vi "TempScanPan.vi"(8 "error in (no error)":errorcluster caption="entrée d'erreur (pas d'erreur)", 11 "LSCI332.lvclass":refnum<class "LSCI332.lvclass">) -> (0 "error out":errorcluster caption="sortie d'erreur", 3 "LSCI332.lvclass Out":refnum<class "LSCI332.lvclass">)   [LabVIEW 2019, in "LSCI332.lvclass"]
uses:
  LSCI332.lvclass
  C:/Programmes Labview/LabScanV1A/DevicesClass/BaseDevice/BaseDevice.lvclass
  BaseDevice/Accessor/GetClassEvent.vi
panel:
  in  "ForceStop":bool
  in  "Wait Stab":bool=TRUE
  in  "Timeout":u32=600 caption="Timeout(s)"
  in  "InRangeTime":i32=300 caption="\"In Range\" Time(s)"
  in  "RangeK":dbl=1.0 min=0.01 max=100.0 step=0.01
  in  "MainProgQEvent":refnum<user-event>
  in  "MainProgQ":refnum<queue>
  in  "Acq":bool
  in  "Boucle(1)":u32(ring) caption="Boucle" items=["Boucle 1", "Boucle 2"]
  in  "Stop":bool
  in  "MiseAJour":bool
  out "Init Program":bool
  # "this MUST labeled with class name"
  # "this MUST be present and labeled \"Stop\""
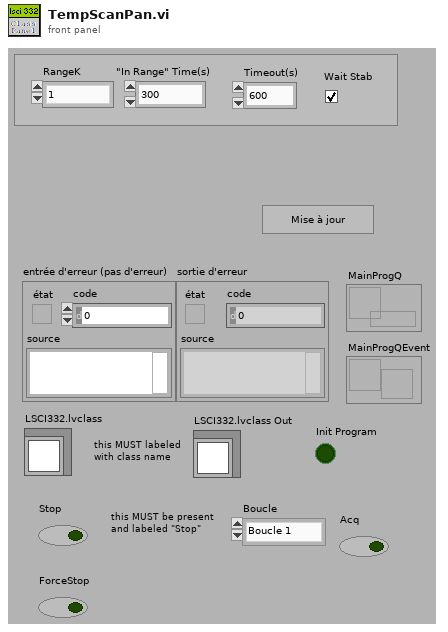
[diagram p1: front panel]
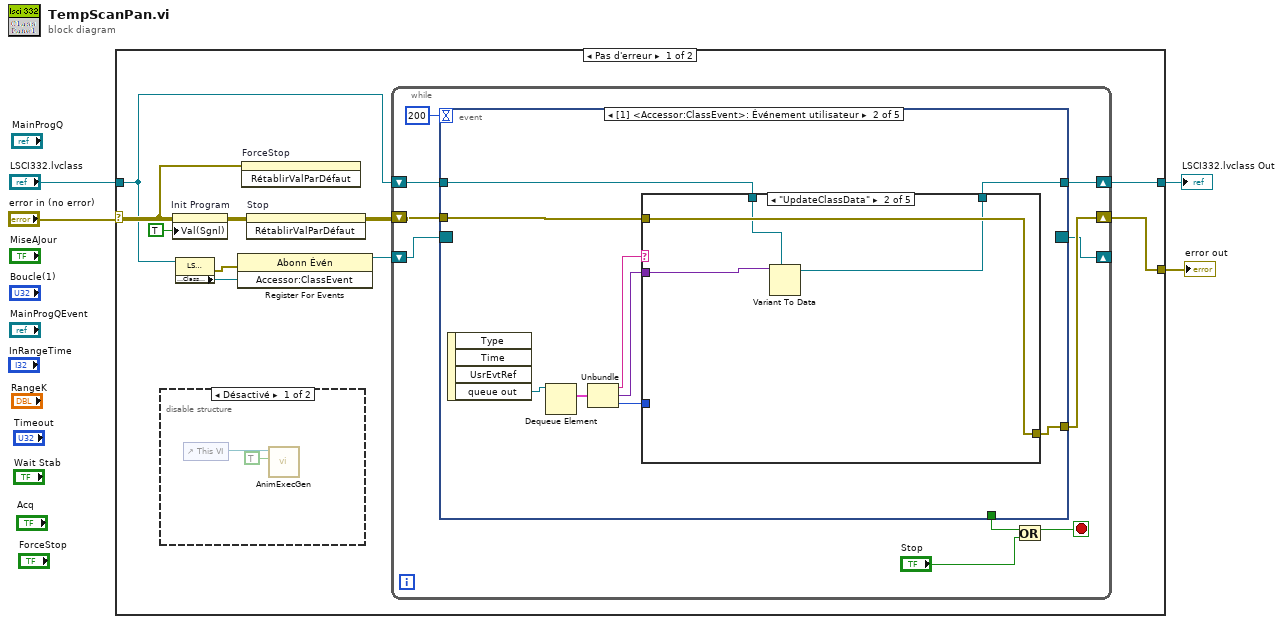
[diagram p0: block diagram]
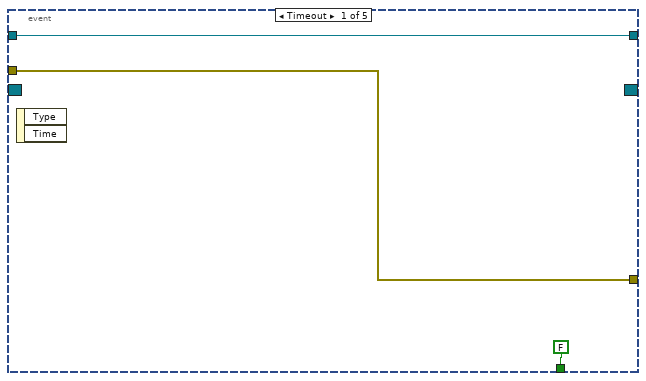
[diagram p3: hidden frame]
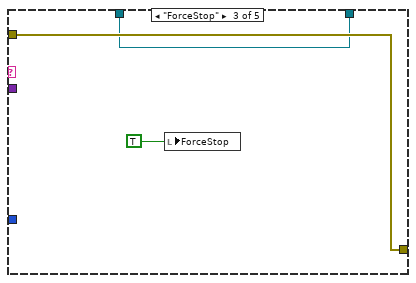
[diagram p5: hidden frame]
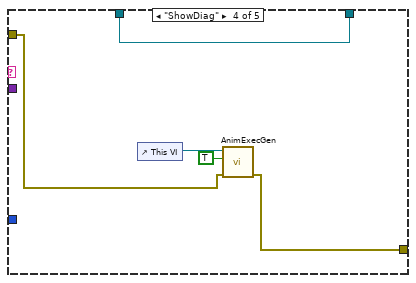
[diagram p6: hidden frame]
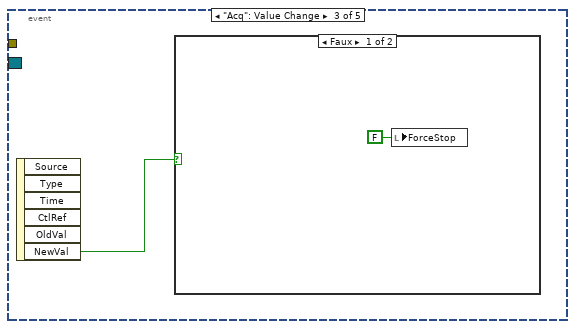
[diagram p8: hidden frame]
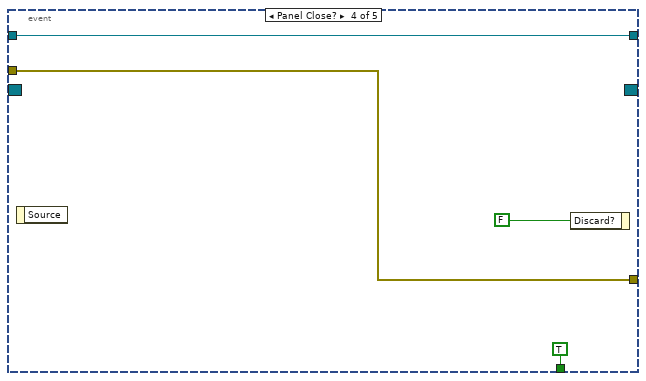
[diagram p10: hidden frame]
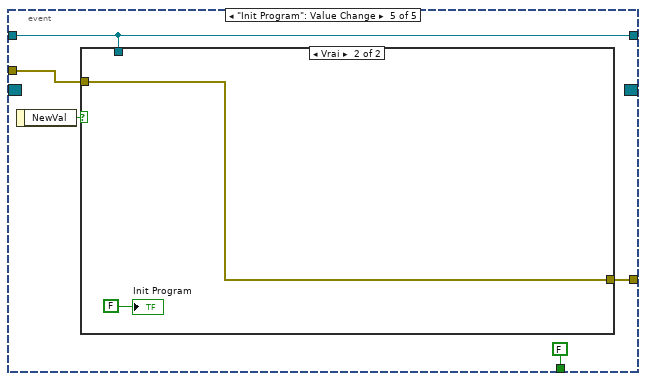
[diagram p11: hidden frame]
diagram:
  n1 = case shown="Pas d'erreur" "error in (no error)" {
    selector: "error in (no error)" -> [w6 w70]
    tunnel: [w14 w70] -> w3
    tunnel: "LSCI332.lvclass" -> [w5 w69]
    tunnel: [w12 w69] -> w1
    frame No Error {
      n2 = disable-structure shown="Désactivé" {
        frame Disabled {
          n3 = control-ref of="This VI"() -> (w15:refnum<vi>)
          n4 = call <userlib>:"AnimExecGen.vi"("Animer l'exécution ?"=TRUE, "ViRef"=w15) -> ()  [unwired: 9 in, 1 out]
        }
        frame Enabled {
        }
      }
      n5 = property on="Init Program" class="Bool (strict)"(error in=w6, "Val(Sgnl)"=TRUE ("Valeur (Signalisation)")) -> (error out=w11:errorcluster)  [unwired: 1 in, 1 out]
      n6 = property class="LSCI332.lvclass"(reference=w5) -> (error out=w9:errorcluster, "Accessor:ClassEvent"=w8:refnum<user-event>)  [unwired: 1 in, 1 out]
      n7 = register-events(error in=w9, w8) -> (reference out=w7:refnum<event-registration>)  [unwired: 1 in, 1 out]
      n8 = invoke on="ForceStop" class="Bool (strict)" method="RétablirValParDéfaut"(error in=w6) -> ()  [unwired: 2 in, 3 out]
      n9 = invoke on="Stop" class="Bool (strict)" method="RétablirValParDéfaut"(error in=w11) -> (error out=w10:errorcluster)  [unwired: 2 in, 2 out]
      n10 = while {
        shift-right: [w24] -> w14
        shift-left: w10 -> [w25]
        shift-right: [w21] -> w12
        shift-left: w5 -> [w23]
        shift-right: [w17] -> _
        shift-left: w7 -> [w18]
        stop <- w20 stop-if-true
        n11 = event shown="[1] <Accessor:ClassEvent>: Événement utilisateur" {
          selector: w18 -> [_ _ _ _ _]
          dyn-events: [_ _ _ _ _] -> w17
          timeout: 200 -> [_ _ _ _ _]
          tunnel: w25 -> [w27 w37 _ w58 w64]
          tunnel: [w27 w31 _ w58 w63] -> w24
          tunnel: w23 -> [w28 w38 _ w57 w61]
          tunnel: [FALSE _ _ TRUE FALSE] -> w22
          tunnel: [w28 w30 _ w57 w61] -> w21
          event Timeout {
            n12 = event-data() -> ()  [unwired: 1 in, 2 out]
          }
          event User Event {
            n13 = event-data() -> ("queue out"=w35:refnum<queue>)  [unwired: 1 in, 3 out]
            n14 = Dequeue Element(queue=w35) -> (element=w36:cluster{"Message":string, "Data":variant, i32})  [unwired: 2 in, 3 out]
            n15 = Unbundle(w36) -> ("Message"=w34:string, "Data"=w33:variant, w32:i32)
            n16 = case shown="\"UpdateClassData\"" w34 {
              tunnel: w37 -> [w40 w44 w47 w49 w53]
              tunnel: w33 -> [_ w43 _ _ _]
              tunnel: w38 -> [w39 w42 w45 w52 w54]
              tunnel: [w39 w41 w45 w52 w54] -> w30
              tunnel: [w40 w44 w47 w48 w53] -> w31
              tunnel: w32 -> [_ _ _ _ _]
              frame Default {
              }
              frame "UpdateClassData" {
                n17 = Variant To Data(type=w42, Variant=w43) -> (data=w41:refnum<class "LSCI332.lvclass">)  [unwired: 1 in, 1 out]
              }
              frame "ForceStop" {
                n18 = local write "ForceStop"(TRUE) -> ()
              }
              frame "ShowDiag" {
                n19 = control-ref of="This VI"() -> (w50:refnum<vi>)
                n20 = call <userlib>:"AnimExecGen.vi"("ErrorIn(No Error)"=w49, "Animer l'exécution ?"=TRUE, "ViRef"=w50) -> ("sortie d'erreur"=w48:errorcluster)  [unwired: 8 in]
              }
              frame "MeasDone" {
              }
            }
          }
          event "Acq": Value Change {
            n21 = event-data() -> ("NewVal"=w55:bool)  [unwired: 1 in, 5 out]
            n22 = case shown="Faux" w55 {
              frame False {
                n23 = local write "ForceStop"(FALSE ("ForceStop")) -> ()
              }
              frame True {
              }
            }
          }
          event Panel Close? {
            n24 = event-data() -> ()  [unwired: 1 in, 1 out]
            n25 = event-data("Discard?"=FALSE ("Rejeter ?")) -> ()  [unwired: 1 in, 1 out]
          }
          event "Init Program": Value Change {
            n26 = event-data() -> ("NewVal"=w65:bool)  [unwired: 1 in]
            n27 = case shown="Vrai" w65 {
              tunnel: w64 -> [w66 w67]
              tunnel: [w66 w67] -> w63
              tunnel: w61 -> [_ _]
              frame False {
              }
              frame True {
                "Init Program" <- FALSE
              }
            }
          }
        }
        n28 = Or(x=w22, y="Stop") -> (x .or. y?=w20:bool)
      }
    }
    frame Error {
    }
  }
  "error out" <- w3
  "LSCI332.lvclass Out" <- w1
